vi "Create Plugins.vi"(8 "error in (no error)":errorcluster, 10 "Plugin Configurations":T1[](array[typedef]) {"Transfer Groups"."Transfers"."channel configurations"."buffer offset" format="%d bytes"}, 11 "Framework in":refnum<class "Framework.lvclass">) -> (0 "error out":errorcluster, 2 "Plugins":refnum<class "Plugin.lvclass">[](array[class]), 3 "Framework out":refnum<class "Framework.lvclass">)   [LabVIEW 2017, in "DSF Core.lvlib" / "Framework.lvclass"]
uses:
  Framework.lvclass
  Configuration/Public/Controls/DSF Engine Plugin Configuration.ctl
  Configuration/Public/Controls/DSF Timing Info.ctl
  Configuration/Public/Controls/DSF Engine Transfer Group Configuration.ctl
  Configuration/Public/Controls/DSF Direction.ctl
  Configuration/Public/Controls/DSF Engine Transfer Configuration.ctl
  Configuration/Public/Controls/DSF Byte Order.ctl
  Configuration/Public/Controls/DSF Engine Channel Configuration.ctl
  Configuration/Public/Controls/DSF Data Type.ctl
  Configuration/Public/Controls/DSF Settings Info.ctl
  Plugin/Plugin.lvclass
  Framework.lvclass/Framework.ctl
  Component Loader/Component Loader.lvclass
  DSF Core.lvlib
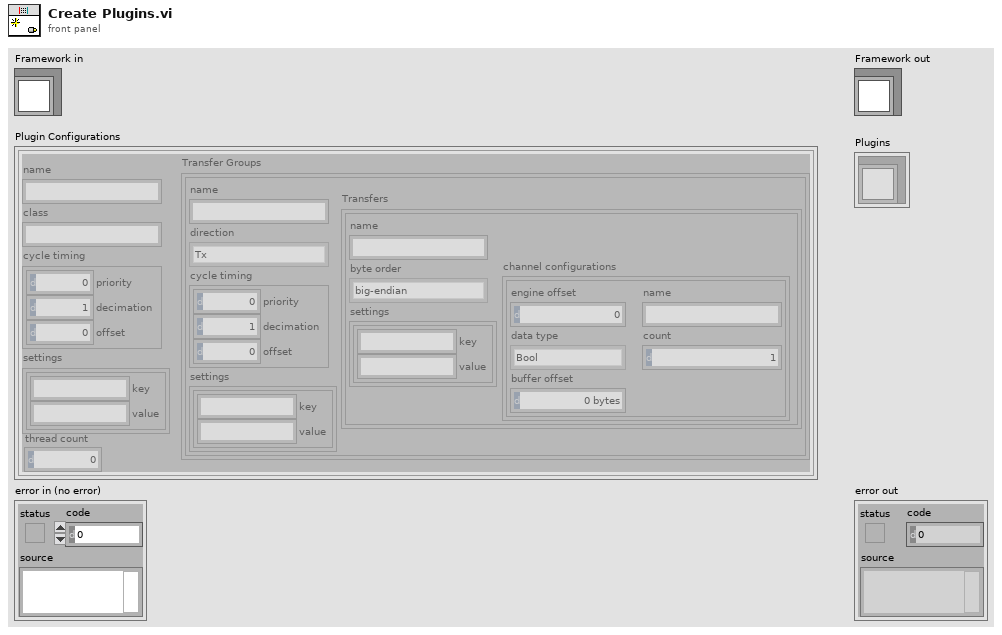
[diagram p1: front panel]
types:
  T1 = typedef "DSF Core.lvlib/DSF Engine Plugin Configuration.ctl" = cluster{"name":string, "class":string, "cycle timing":T2, "Transfer Groups":T3[], "settings":T9, "thread count":i32}
  T2 = typedef "DSF Core.lvlib/DSF Timing Info.ctl" = cluster{"priority":u64, "decimation":u64, "offset":u64}
  T3 = typedef "DSF Core.lvlib/DSF Engine Transfer Group Configuration.ctl" = cluster{"name":string, "direction":T4, "cycle timing":T2, "Transfers":T5[], "settings":T9}
  T4 = typedef "DSF Core.lvlib/DSF Direction.ctl" = enum8{"Tx", "Rx"}
  T5 = typedef "DSF Core.lvlib/DSF Engine Transfer Configuration.ctl" = cluster{"name":string, "byte order":T6, "channel configurations":T7[], "settings":T9}
  T6 = typedef "DSF Core.lvlib/DSF Byte Order.ctl" = enum8{"big-endian", "little-endian"}
  T7 = typedef "DSF Core.lvlib/DSF Engine Channel Configuration.ctl" = cluster{"engine offset":u64, "name":string, "data type":T8, "count":u64, "buffer offset":u64}
  T8 = typedef "DSF Core.lvlib/DSF Data Type.ctl" = enum8{"Bool", "SGL", "DBL", "I8", "I16", "I32", "I64", "U8", "U16", "U32", "U64"}
  T9 = typedef "DSF Core.lvlib/DSF Settings Info.ctl" = cluster{"key":string, "value":string}[]
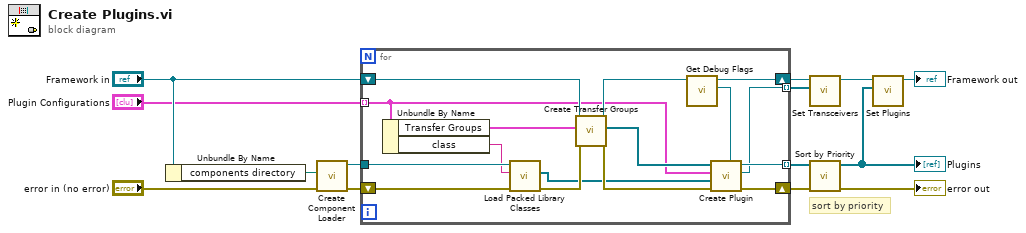
[diagram p0: block diagram]
diagram:
  # "sort by priority"
  n1 = Unbundle By Name("Framework in") -> ("components directory"=w4:path)
  n2 = call "Create Component Loader.vi"("error in (no error)"="error in (no error)", "components directory"=w4) -> ("error out"=w5:errorcluster, "Component Loader out"=w7:refnum<class "Component Loader.lvclass">)  [unwired: 8 in]
  n3 = for {
    shift-right: [w28] -> w13
    shift-left: w5 -> [w18]
    shift-right: [w24] -> w9
    shift-left: "Framework in" -> [w27]
    tunnel: "Plugin Configurations" -> [w16] mode=indexing
    tunnel: [w26] -> w11 mode=indexing
    tunnel: w7 -> [w23]
    tunnel: [w22] -> w6 mode=indexing
    n4 = Unbundle By Name(w16) -> ("Transfer Groups"=w17:T3[], "class"=w15:string)
    n5 = call "Load Packed Library Classes.vi"("error in (no error)"=w18, "packed library name"=w15, "Component Loader in"=w23) -> ("error out"=w29:errorcluster, "objects"=w20:refnum<class>[])  [unwired: 6 in, 1 out]
    n6 = call "Create Transfer Groups.vi"("error in (no error)"=w29, "Transfer Group Configurations"=w17, "Framework in"=w27) -> ("error out"=w30:errorcluster, "Transfer Groups"=w19:refnum<class "Transfer Group.lvclass">[], "Framework out"=w25:refnum<class "Framework.lvclass">)  [unwired: 6 in]
    n7 = call "Get Debug Flags.vi"("Framework in"=w25) -> ("Debug Flags"=w21:refnum<class "Debug Flags.lvclass">, "Framework out"=w24:refnum<class "Framework.lvclass">)  [unwired: 9 in]
    n8 = call "Create Plugin.vi"("Debug Flags"=w21, "error in (no error)"=w30, "component classes"=w20, "Plugin Configuration"=w16, "Transfer Groups"=w19) -> ("error out"=w28:errorcluster, "Transceiver"=w22:refnum<class "Transceiver.lvclass">, "Plugin out"=w26:refnum<class "Plugin.lvclass">)  [unwired: 3 in, 1 out]
  }
  n9 = call "Set Transceivers.vi"("Transceivers"=w6, "Framework in"=w9) -> ("Framework out"=w8:refnum<class "Framework.lvclass">)  [unwired: 9 in]
  n10 = call "Sort by Priority.vi"("error in (no error)"=w13, "Plugins in"=w11) -> ("error out"=→"error out":errorcluster, "Plugins out"=w10:refnum<class "Plugin.lvclass">[])  [unwired: 8 in]
  "Plugins" <- w10
  n11 = call "Set Plugins.vi"("Plugins"=w10, "Framework in"=w8) -> ("Framework out"=→"Framework out":refnum<class "Framework.lvclass">)  [unwired: 9 in]
